vi "isolateNextStringElement.vi"(8 "error in (no error)":errorcluster, 9 "Final Delimiter":T1, 10 "inputString":string, 11 "TEI9150 in":refnum<class "Tovey9150.lvclass">) -> (0 "error out":errorcluster, 1 "remainingString":string, 2 "extractedSegment":string, 3 "TEI9150 out":refnum<class "Tovey9150.lvclass">)   [LabVIEW 2015, in "Tovey9150.lvclass"]
uses:
  Tovey9150.lvclass
  <userlib>/Common/ILC/ILCModelTypedefs/FinalDelimiter.ctl
  <userlib>/Common/ILC/ILCModelTypedefs/ILCModelTypedefs.lvlib
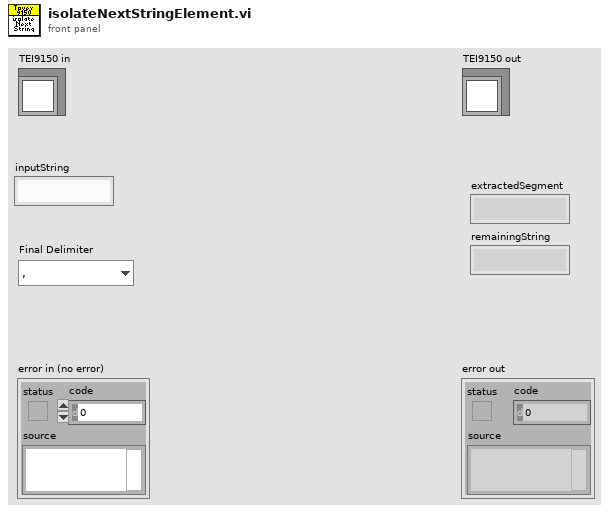
[diagram p1: front panel]
types:
  T1 = typedef "ILCCommon.lvlib/ILCModelTypedefs.lvlib/FinalDelimiter.ctl" = enum16{",", "<CR><LF>"}
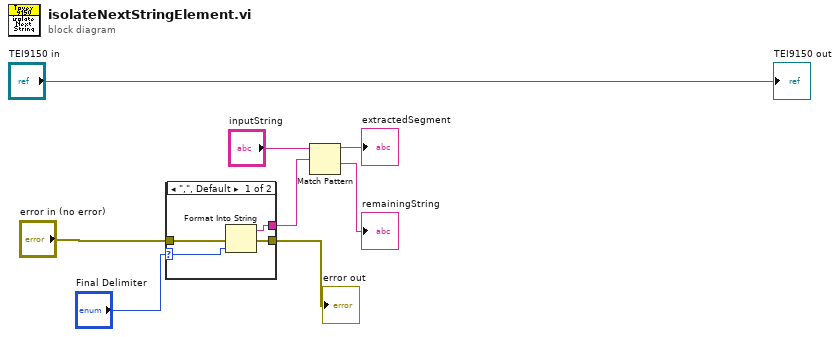
[diagram p0: block diagram]
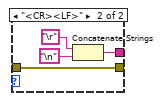
[diagram p2: hidden frame]
diagram:
  n1 = case shown="\",\", Default" "Final Delimiter" {
    selector: "Final Delimiter" -> [w12 _]
    tunnel: [w11 w14] -> w6
    tunnel: "error in (no error)" -> [w10 w13]
    tunnel: [w9 w13] -> w1
    frame ",", Default {
      n2 = Format Into String(error in=w10, w12) -> (resulting string=w11:string, error out=w9:errorcluster)  [unwired: 2 in]
    }
    frame "<CR><LF>" {
      n3 = Concatenate Strings("\r", "\n") -> (w14:string)
    }
  }
  "error out" <- w1
  n4 = Match Pattern(string="inputString", regular expression=w6) -> (before substring=→"extractedSegment":string, after substring=→"remainingString":string)  [unwired: 1 in, 2 out]
  "TEI9150 out" <- "TEI9150 in"
